vi "CRYGet Tree Step DispNo.vi"(0 "SequenceTree":refnum<vi>, 11 "Active Item Tag":string) -> (4 "reference out":refnum<vi>, 15 "Active Cell String1":string)   [LabVIEW 2013]
panel:
  out "error out":errorcluster
  in  "error in (no error)":errorcluster
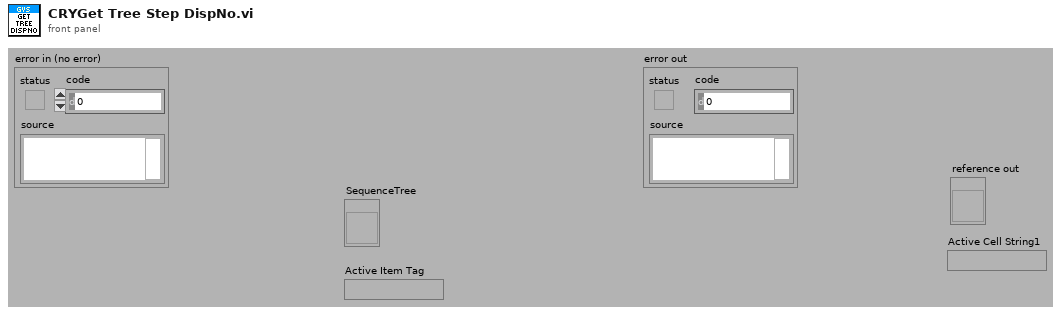
[diagram p1: front panel]
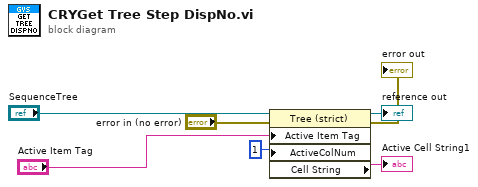
[diagram p0: block diagram]
diagram:
  n1 = property class="Tree (strict)"(reference="SequenceTree", error in="error in (no error)", "Active Item Tag"="Active Item Tag", "ActiveColNum"=1 ("Active Cell:Active Column Number")) -> (reference out=→"reference out":refnum<vi>, error out=→"error out":errorcluster, "Cell String"=→"Active Cell String1":string)
